vi "Alternating LEDs.vi"() -> ()   [LabVIEW 2015]
panel:
  in  "Boolean":bool
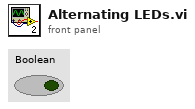
[diagram p1: front panel]
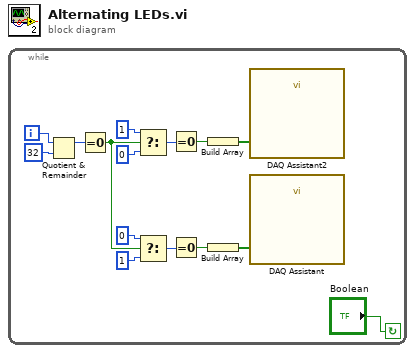
[diagram p0: block diagram]
diagram:
  n1 = while {
    i -> [w9]
    stop <- "Boolean" continue-if-true
    n2 = Quotient & Remainder(x=w9, y=32) -> (x-y*floor(x/y)=w8:i32)  [unwired: 1 out]
    n3 = Equal To 0?(x=w8) -> (x = 0?=w7:bool)
    n4 = Select(t=1, s=w7, f=0) -> (s? t:f=w15:i32)
    n5 = Select(t=0, s=w7, f=1) -> (s? t:f=w12:i32)
    n6 = Equal To 0?(x=w15) -> (x = 0?=w3:bool)
    n7 = Equal To 0?(x=w12) -> (x = 0?=w1:bool)
    n8 = Build Array(w3) -> (w4:bool[])
    n9 = Build Array(w1) -> (w2:bool[])
    n10 = call "DAQ Assistant2"("data"=w4) -> ()  [unwired: 17 in, 2 out]
    n11 = call "DAQ Assistant"("data"=w2) -> ()  [unwired: 17 in, 2 out]
  }
